vi "bead_dropper_Gadi.vi"() -> ()   [LabVIEW 2016]
uses:
  <vilib>/Instr/_visa.llb/VISA Open Access Mode.ctl
  <instrlib>/Agilent 33XXX Series/Agilent 33XXX Series.lvlib
panel:
  in  "seconds between steps":u32=5
  out "Last Voltage":dbl=17.5
  in  "stop":bool
  in  "Stop  Frequency (kHz)":dbl=300.0 format="%#.6g"
  in  "Start Frequency (kHz)":dbl=100.0 format="%#.6g"
  in  "Sweep Time (s)":dbl=0.1 format="%#.6g"
  in  "Step size (V)":dbl=0.3
  in  "Start Voltage (V)":dbl=16.0
  in  "Number of steps":i32=30
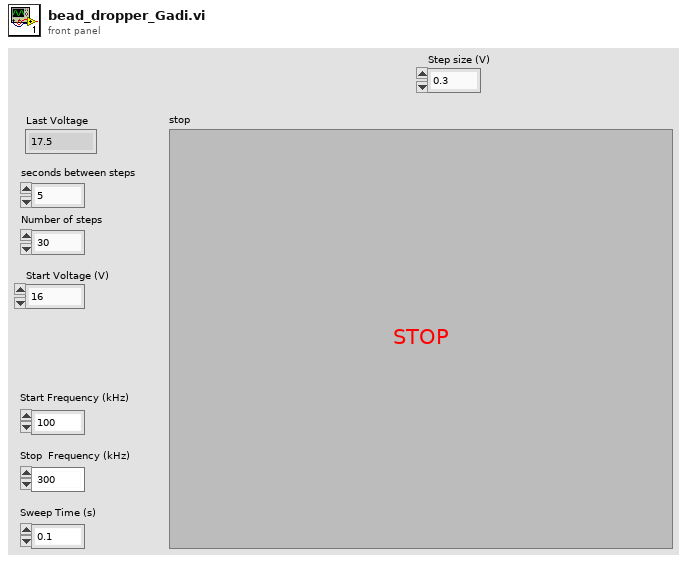
[diagram p1: front panel]
types:
  T1 = typedef "VISA Open Access Mode.ctl" = u32
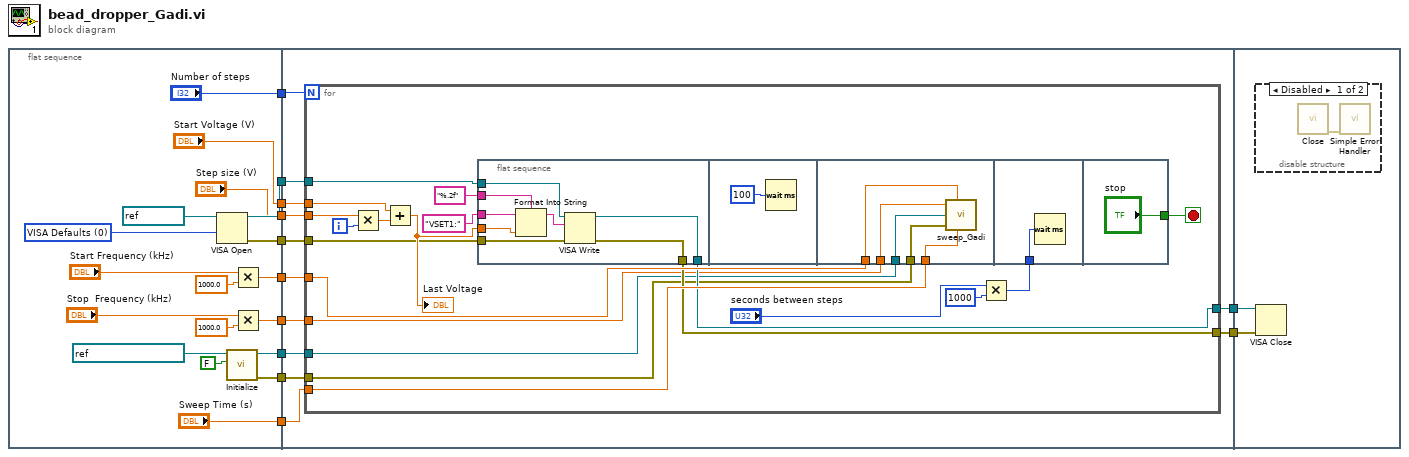
[diagram p0: block diagram]
diagram:
  n1 = flat-sequence {
    tunnel: ["Number of steps"] -> w12
    tunnel: [w25] -> w11
    tunnel: [w24] -> w10
    tunnel: [w19] -> w9
    tunnel: [w18] -> w8
    tunnel: ["Sweep Time (s)"] -> w7
    tunnel: ["Start Voltage (V)"] -> w6
    tunnel: ["Step size (V)"] -> w5
    tunnel: [w14] -> w2
    tunnel: [w13] -> w1
    tunnel: w12 -> [w42]
    tunnel: w11 -> [w41]
    tunnel: w10 -> [w40]
    tunnel: w9 -> [w39]
    tunnel: w8 -> [w38]
    tunnel: w7 -> [w37]
    tunnel: w6 -> [w36]
    tunnel: w5 -> [w35]
    tunnel: [w34] -> w4
    tunnel: [w33] -> w3
    tunnel: w2 -> [w32]
    tunnel: w1 -> [w31]
    tunnel: w4 -> [w80]
    tunnel: w3 -> [w79]
    frame #0 {
      w27 = T1 0 items=["VISA Defaults"=0, "Exclusive Lock"=1, "Load Configured Settings"=4] ("Access Mode")
      n2 = VISA Open(access mode=w27, VISA resource name=refnum<visa-resource-name> "COM4") -> (VISA resource name=w25:refnum<visa-resource-name>, error out=w24:errorcluster)  [unwired: 3 in]
      n3 = call <instrlib>:"Initialize.vi"("ID Query (True)"=FALSE, "VISA resource name"=refnum<visa-resource-name> "K-33511B-03409") -> ("error out"=w14:errorcluster, "VISA resource name out"=w13:refnum<visa-resource-name>)  [unwired: 8 in]
      n4 = Multiply(x="Start Frequency (kHz)", y=1000.0) -> (x*y=w18:dbl)
      n5 = Multiply(x="Stop  Frequency (kHz)", y=1000.0) -> (x*y=w19:dbl)
    }
    frame #1 {
      n6 = for {
        N: w42 -> [_]
        tunnel: w36 -> [w62]
        tunnel: w35 -> [w61]
        tunnel: w38 -> [w54]
        tunnel: w37 -> [w55]
        tunnel: w41 -> [w53]
        tunnel: [w52] -> w33
        tunnel: w40 -> [w51]
        tunnel: [w50] -> w34
        tunnel: w39 -> [w45]
        tunnel: w32 -> [w44]
        tunnel: w31 -> [w43]
        i -> [w60]
        stop <- w46 stop-if-true
        n7 = Multiply(x=w61, y=w60) -> (x*y=w59:dbl)
        n8 = Add(x=w62, y=w59) -> (x+y=w58:dbl)
        "Last Voltage" <- w58
        n9 = flat-sequence {
          tunnel: w58 -> [w70]
          tunnel: "VSET1:" ("write buffer") -> [w69]
          tunnel: "%.2f" ("format string") -> [w68]
          tunnel: w53 -> [w67]
          tunnel: [w66] -> w52
          tunnel: w51 -> [w65]
          tunnel: [w64] -> w50
          tunnel: w55 -> [w72]
          tunnel: w54 -> [w73]
          tunnel: w45 -> [w74]
          tunnel: w44 -> [w76]
          tunnel: w43 -> [w75]
          tunnel: w47 -> [w77]
          tunnel: ["stop"] -> w46
          frame #0 {
            n10 = Format Into String(format string=w68, initial string=w69, w70) -> (resulting string=w63:string)  [unwired: 1 in, 1 out]
            n11 = VISA Write(VISA resource name=w67, write buffer=w63, error in (no error)=w65) -> (VISA resource name out=w66:refnum<visa-resource-name>, error out=w64:errorcluster)  [unwired: 1 out]
          }
          frame #1 {
            n12 = Wait (ms)(milliseconds to wait=u32 100) -> ()  [unwired: 1 out]
          }
          frame #2 {
            n13 = call "sweep_Gadi.vi"("Stop  Frequency (1000.0 Hz)"=w74, "Start Frequency (100.0 Hz)"=w73, "VISA resource name in"=w75, "error in (no error)"=w76, "Sweep Time (1.00 s)"=w72) -> ()  [unwired: 5 in]
          }
          frame #3 {
            n14 = Wait (ms)(milliseconds to wait=w77) -> ()  [unwired: 1 out]
          }
          frame #4 {
          }
        }
        n15 = Multiply(x="seconds between steps", y=u32 1000) -> (x*y=w47:u32)
      }
    }
    frame #2 {
      n16 = disable-structure shown="Disabled" {
        frame Disabled {
          n17 = call <instrlib>:"Close.vi"() -> ("error out"=w81:errorcluster)  [unwired: 11 in]
          n18 = call <vilib>:"Simple Error Handler.vi"("error in (no error)"=w81) -> ()  [unwired: 4 in, 5 out]
        }
        frame Enabled {
        }
      }
      n19 = VISA Close(VISA resource name=w79, error in (no error)=w80) -> ()  [unwired: 1 out]
    }
  }
